vi "Dialog Box.vi"(8 "error in (no error)":errorcluster, 11 "Dialog_2Buttons in":refnum<class "Dialog_TwoButtons.lvclass">) -> (0 "error out":errorcluster, 1 "timed out?":bool, 2 "Selection":string, 3 "Dialog_2Buttons out":refnum<class "Dialog_TwoButtons.lvclass">)   [LabVIEW 2012, in "Dialog_TwoButtons.lvlib" / "Dialog_TwoButtons.lvclass"]
doc: "This VI contains the code for the dialog box.\nOverride this VI to provide more functionality or to create your own application-specific dialog box."
uses:
  Dialog_TwoButtons.lvclass
  Fading/_Fade In(I32).vi
panel:
  out "String":string
  in  "Cancel Button":bool
  in  "OK Button":bool
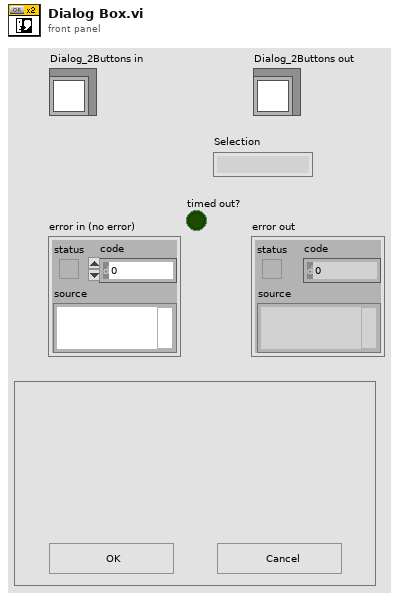
[diagram p1: front panel]
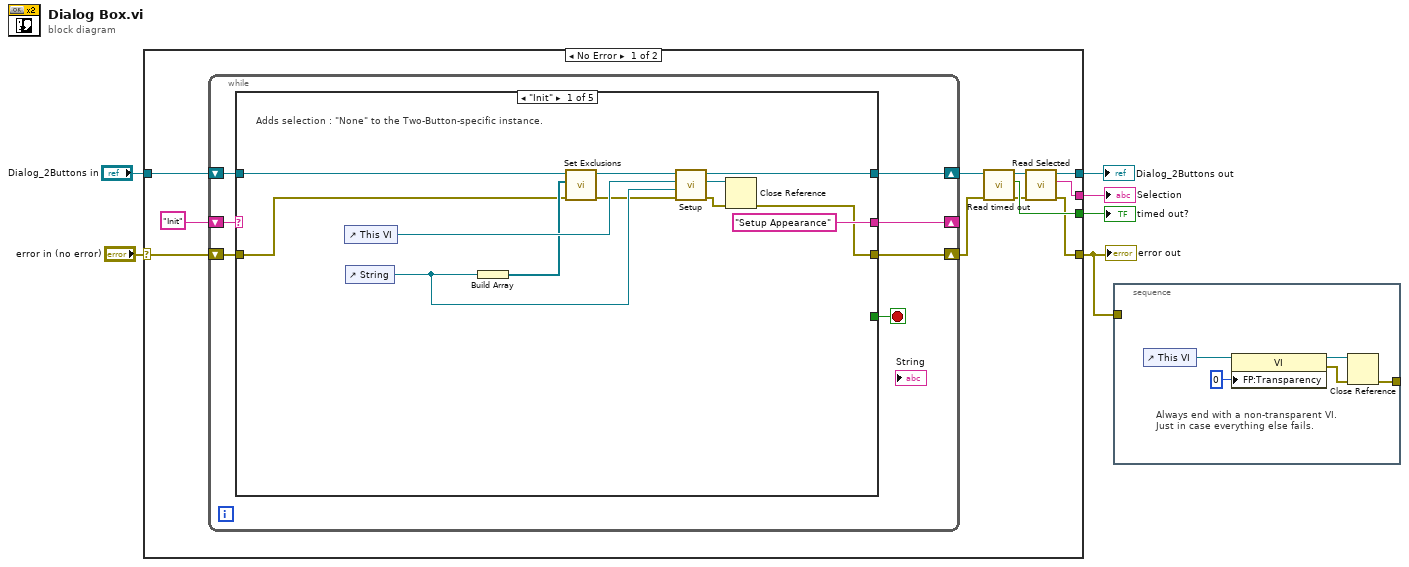
[diagram p0: block diagram]
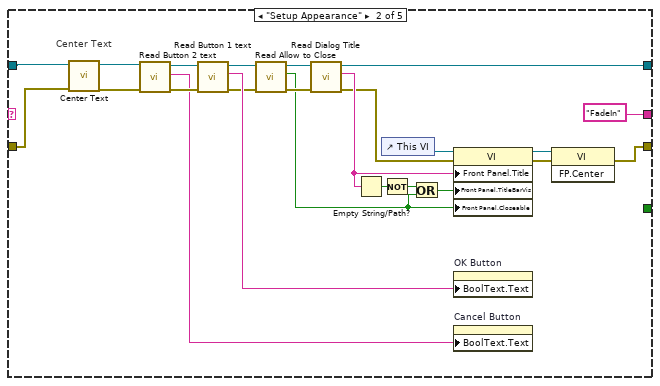
[diagram p2: hidden frame]
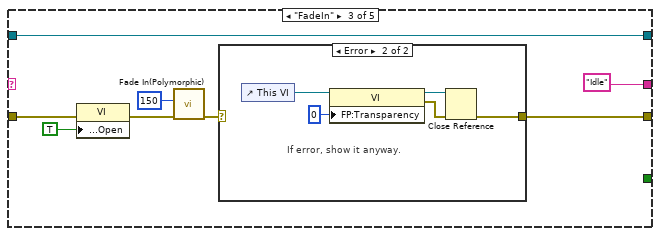
[diagram p3: hidden frame]
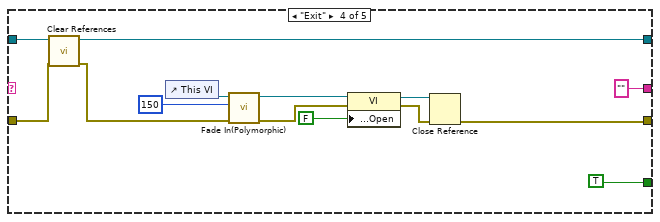
[diagram p5: hidden frame]
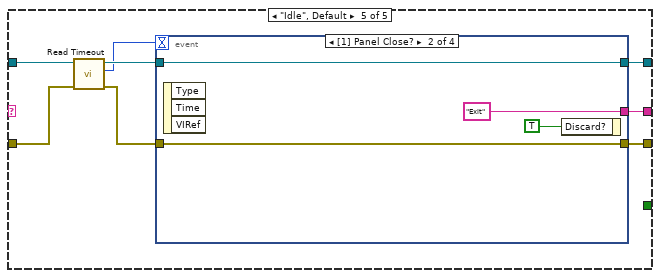
[diagram p6: hidden frame]
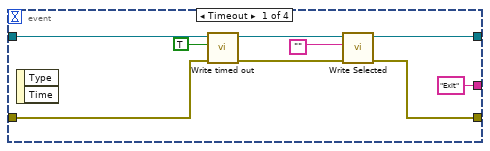
[diagram p7: hidden frame]
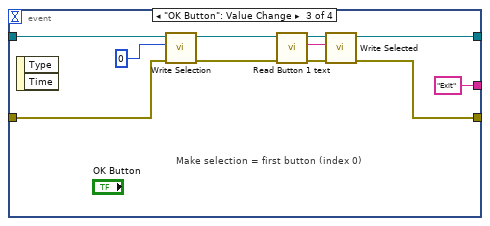
[diagram p8: hidden frame]
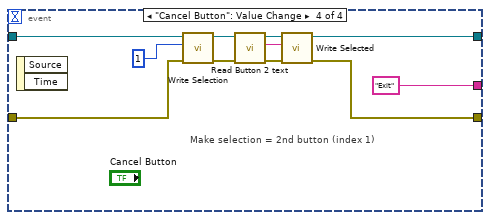
[diagram p9: hidden frame]
diagram:
  n1 = case shown="No Error" "error in (no error)" {
    selector: "error in (no error)" -> [w16 w133]
    tunnel: [w8 w133] -> w1
    tunnel: [w10 w132] -> w6
    tunnel: "Dialog_2Buttons in" -> [w17 w132]
    tunnel: [w12 _] -> w3
    tunnel: [w9 _] -> w2
    frame No Error {
      n2 = while {
        shift-right: [w19] -> _
        shift-left: "Init" -> [w20]
        shift-right: [w24] -> w14
        shift-left: w17 -> [w23]
        shift-right: [w22] -> w13
        shift-left: w16 -> [w21]
        stop <- w18 stop-if-true
        n3 = case shown="\"Init\"" w20 {
          tunnel: [w30 w49 w68 w77 w89] -> w24
          tunnel: w23 -> [w28 w47 w68 w78 w94]
          tunnel: [w29 w55 w64 w80 w96] -> w22
          tunnel: w21 -> [w27 w44 w62 w76 w91]
          tunnel: ["Setup Appearance" "FadeIn" "Idle" "" w95] -> w19
          tunnel: [_ _ _ TRUE _] -> w18
          frame "Init" {
            # "Adds selection : \"None\" to the Two-Button-specific instance."
            n4 = control-ref of="This VI"() -> (w35:refnum<vi>)
            n5 = control-ref of="String"() -> (w31:refnum<vi>)
            n6 = Build Array(w31) -> (w33:refnum<vi>[])
            n7 = call-dynamic "Set Exclusions.vi"("error in (no error)"=w27, "Exclusions"=w33, "Dialog in"=w28) -> ("error out"=w25:errorcluster, "Dialog out"=w26:refnum<class "Dialog_TwoButtons.lvclass">)  [unwired: 7 out]
            n8 = call-dynamic "Setup.vi"("error in (no error)"=w25, "Str Refnum"=w31, "VI Reference"=w35, "Dialog_TwoButtons in"=w26) -> ("error out"=w34:errorcluster, "VI reference (dup)"=w32:refnum<vi>, "Dialog_TwoButtons out"=w30:refnum<class "Dialog_TwoButtons.lvclass">)  [unwired: 5 out]
            n9 = Close Reference(reference=w32, error in (no error)=w34) -> (error out=w29:errorcluster)
          }
          frame "Setup Appearance" {
            # "Center Text"
            n10 = call-dynamic "Center Text.vi"("error in (no error)"=w44, "Dialog in"=w47) -> ("error out"=w45:errorcluster, "Dialog out"=w46:refnum<class "Dialog_TwoButtons.lvclass">)  [unwired: 8 out]
            n11 = call-dynamic "Read Button 2 text.vi"("error in (no error)"=w45, "Dialog_2Buttons.lvclass in"=w46) -> ("error out"=w52:errorcluster, "Button #2 text"=w50:string, "Dialog_2Buttons.lvclass out"=w53:refnum<class "Dialog_TwoButtons.lvclass">)  [unwired: 7 out]
            n12 = call-dynamic "Read Button 1 text.vi"("error in (no error)"=w52, "Dialog_2Buttons.lvclass in"=w53) -> ("error out"=w41:errorcluster, "Button #1 text"=w51:string, "Dialog_2Buttons.lvclass out"=w43:refnum<class "Dialog_TwoButtons.lvclass">)  [unwired: 7 out]
            n13 = call-dynamic "Read Allow to Close.vi"("error in (no error)"=w41, "Dialog.lvclass in"=w43) -> ("error out"=w40:errorcluster, "Allow to close?"=w39:bool, "Dialog.lvclass out"=w42:refnum<class "Dialog_TwoButtons.lvclass">)  [unwired: 7 out]
            n14 = call-dynamic "Read Dialog Title.vi"("error in (no error)"=w40, "Dialog in"=w42) -> ("error out"=w48:errorcluster, "Dialog Title"=w54:string, "Dialog out"=w49:refnum<class "Dialog_TwoButtons.lvclass">)  [unwired: 7 out]
            n15 = Empty String/Path?(string/path=w54) -> (empty?=w58:bool)
            n16 = control-ref of="This VI"() -> (w59:refnum<vi>)
            n17 = Not(x=w58) -> (.not. x?=w38:bool)
            n18 = Or(x=w38, y=w39) -> (x .or. y?=w37:bool)
            n19 = property class="VI"(reference=w59, error in=w48, "Front Panel.Title"=w54, "Front Panel.TitleBarVis"=w37, "Front Panel.Closeable"=w39) -> (reference out=w57:refnum<vi>, error out=w56:errorcluster)
            n20 = property on="OK Button" class="Bool"("BoolText.Text"=w51) -> ()  [unwired: 2 in, 2 out]
            n21 = property on="Cancel Button" class="Bool"("BoolText.Text"=w50) -> ()  [unwired: 2 in, 2 out]
            n22 = invoke class="VI" method="FP.Center"(reference=w57, error in=w56) -> (error out=w55:errorcluster)  [unwired: 1 in, 2 out]
          }
          frame "FadeIn" {
            n23 = property class="VI"(error in=w62, "Front Panel.Open"=TRUE ("Front Panel Window:Open")) -> (error out=w61:errorcluster)  [unwired: 1 in, 1 out]
            n24 = call-poly "Fade In(Polymorphic).vi"("error in"=w61, "Fade time (ms)"=150) -> ("error out"=w65:errorcluster)  [unwired: 2 in, 7 out]
            n25 = case shown="Error" w65 {
              selector: w65 -> [w69 _]
              tunnel: [w69 w70] -> w64
              frame No Error {
              }
              frame Error {
                # "If error, show it anyway."
                n26 = control-ref of="This VI"() -> (w72:refnum<vi>)
                n27 = property class="VI"(reference=w72, "FP:Transparency"=u8 0 ("Front Panel Window:Transparency")) -> (reference out=w73:refnum<vi>, error out=w74:errorcluster)  [unwired: 1 in]
                n28 = Close Reference(reference=w73, error in (no error)=w74) -> (error out=w70:errorcluster)
              }
            }
          }
          frame "Exit" {
            n29 = call-dynamic "Clear References.vi"("error in (no error)"=w76, "Dialog in"=w78) -> ("error out"=w75:errorcluster, "Dialog out"=w77:refnum<class "Dialog_TwoButtons.lvclass">)  [unwired: 8 out]
            n30 = control-ref of="This VI"() -> (w79:refnum<vi>)
            n31 = call-poly "Fade In(Polymorphic).vi"("error in"=w75, "Fade time (ms)"=150, "VI Reference (calling VI)"=w79) -> ("error out"=w81:errorcluster, "dup VI Reference"=w82:refnum<vi>)  [unwired: 1 in, 6 out]
            n32 = property class="VI"(reference=w82, error in=w81, "Front Panel.Open"=FALSE ("Front Panel Window:Open")) -> (reference out=w84:refnum<vi>, error out=w83:errorcluster)
            n33 = Close Reference(reference=w84, error in (no error)=w83) -> (error out=w80:errorcluster)
          }
          frame "Idle", Default {
            n34 = call-dynamic "Read Timeout.vi"("error in (no error)"=w91, "Dialog.lvclass in"=w94) -> ("error out"=w90:errorcluster, "Timeout"=w92:i32, "Dialog.lvclass out"=w93:refnum<class "Dialog_TwoButtons.lvclass">)  [unwired: 7 out]
            n35 = event shown="[1] Panel Close?" {
              selector: _ -> [_ _ _ _]
              dyn-events: _ -> [_ _ _ _]
              timeout: w92 -> [_ _ _ _]
              tunnel: w93 -> [w104 w109 w118 w129]
              tunnel: [w98 w108 w111 w121] -> w96
              tunnel: w90 -> [w102 w108 w117 w128]
              tunnel: ["Exit" "Exit" "Exit" "Exit"] -> w95
              tunnel: [w97 w109 w113 w125] -> w89
              event Timeout {
                n36 = event-data() -> ()  [unwired: 3 out]
                n37 = call-dynamic "Write timed out.vi"("error in (no error)"=w102, "timed out?"=TRUE, "Dialog.lvclass in"=w104) -> ("error out"=w99:errorcluster, "Dialog.lvclass out"=w101:refnum<class "Dialog_TwoButtons.lvclass">)  [unwired: 7 out]
                n38 = call-dynamic "Write Selected.vi"("error in (no error)"=w99, "Selected"="", "Dialog.lvclass in"=w101) -> ("error out"=w98:errorcluster, "Dialog.lvclass out"=w97:refnum<class "Dialog_TwoButtons.lvclass">)  [unwired: 7 out]
              }
              event Panel Close? {
                n39 = event-data() -> ()  [unwired: 4 out]
                n40 = event-data("Discard?"=TRUE) -> ()  [unwired: 1 in, 1 out]
              }
              event "OK Button": Value Change {
                # "Make selection = first button (index 0)"
                n41 = event-data() -> ()  [unwired: 3 out]
                n42 = call-dynamic "Write Selection.vi"("error in (no error)"=w117, "Selection (-1: none)"=i8 0, "Dialog_2Buttons.lvclass in"=w118) -> ("error out"=w115:errorcluster, "Dialog_2Buttons.lvclass out"=w116:refnum<class "Dialog_TwoButtons.lvclass">)  [unwired: 7 out]
                n43 = call-dynamic "Read Button 1 text.vi"("error in (no error)"=w115, "Dialog_2Buttons.lvclass in"=w116) -> ("error out"=w112:errorcluster, "Button #1 text"=w110:string, "Dialog_2Buttons.lvclass out"=w114:refnum<class "Dialog_TwoButtons.lvclass">)  [unwired: 7 out]
                n44 = call-dynamic "Write Selected.vi"("error in (no error)"=w112, "Selected"=w110, "Dialog.lvclass in"=w114) -> ("error out"=w111:errorcluster, "Dialog.lvclass out"=w113:refnum<class "Dialog_TwoButtons.lvclass">)  [unwired: 7 out]
              }
              event "Cancel Button": Value Change {
                # "Make selection = 2nd button (index 1)"
                n45 = event-data() -> ()  [unwired: 3 out]
                n46 = call-dynamic "Write Selection.vi"("error in (no error)"=w128, "Selection (-1: none)"=i8 1, "Dialog_2Buttons.lvclass in"=w129) -> ("error out"=w124:errorcluster, "Dialog_2Buttons.lvclass out"=w127:refnum<class "Dialog_TwoButtons.lvclass">)  [unwired: 7 out]
                n47 = call-dynamic "Read Button 2 text.vi"("error in (no error)"=w124, "Dialog_2Buttons.lvclass in"=w127) -> ("error out"=w123:errorcluster, "Button #2 text"=w122:string, "Dialog_2Buttons.lvclass out"=w126:refnum<class "Dialog_TwoButtons.lvclass">)  [unwired: 7 out]
                n48 = call-dynamic "Write Selected.vi"("error in (no error)"=w123, "Selected"=w122, "Dialog.lvclass in"=w126) -> ("error out"=w121:errorcluster, "Dialog.lvclass out"=w125:refnum<class "Dialog_TwoButtons.lvclass">)  [unwired: 7 out]
              }
            }
          }
        }
      }
      n49 = call-dynamic "Read timed out.vi"("error in (no error)"=w13, "Dialog.lvclass in"=w14) -> ("error out"=w7:errorcluster, "timed out?"=w12:bool, "Dialog.lvclass out"=w11:refnum<class "Dialog_TwoButtons.lvclass">)  [unwired: 7 out]
      n50 = call-dynamic "Read Selected.vi"("error in (no error)"=w7, "Dialog.lvclass in"=w11) -> ("error out"=w8:errorcluster, "Selected"=w9:string, "Dialog.lvclass out"=w10:refnum<class "Dialog_TwoButtons.lvclass">)  [unwired: 7 out]
    }
    frame Error {
    }
  }
  "error out" <- w1
  "Dialog_2Buttons out" <- w6
  "timed out?" <- w3
  "Selection" <- w2
  n51 = stacked-sequence {
    tunnel: w1 -> [_]
    tunnel: [w134] -> _
    frame #0 {
      # "Always end with a non-transparent VI.\nJust in case everything else fails."
      n52 = control-ref of="This VI"() -> (w137:refnum<vi>)
      n53 = property class="VI"(reference=w137, "FP:Transparency"=u8 0 ("Front Panel Window:Transparency")) -> (reference out=w136:refnum<vi>, error out=w135:errorcluster)  [unwired: 1 in]
      n54 = Close Reference(reference=w136, error in (no error)=w135) -> (error out=w134:errorcluster)
    }
  }
